vi "KGN Get Pump Massflow.vi"(7 "scaling":dbl=1000000.0, 8 "Fehler (Eingang, kein Fehler)":errorcluster, 9 "Info Cluster":T2, 10 "VISA-Referenz (Eingang)":refnum<visa-resource-name>, 11 "device (Eingang)":u32) -> (0 "Fehler (Ausgang)":errorcluster, 1 "Info Cluster out":T2, 2 "VISA-Referenz (Ausgang)":refnum<visa-resource-name>, 3 "dup device (Ausgang)":u32, 4 "Pump MassFlow-Cluster":T1(array[cluster]), 6 "Kommandos gesendet":string)   [LabVIEW 2020, in "Linearisierung v2.lvlib" / "Gasteiler.lvlib" / "HovaCAL_Interface.lvlib" / "KGN.lvlib" / "KGN GUI Get.lvlib"]
uses:
  KGN GUI Get.lvlib
  Controls/Info Cluster.ctl
  get/get.lvlib
  Controls/Controls.lvlib
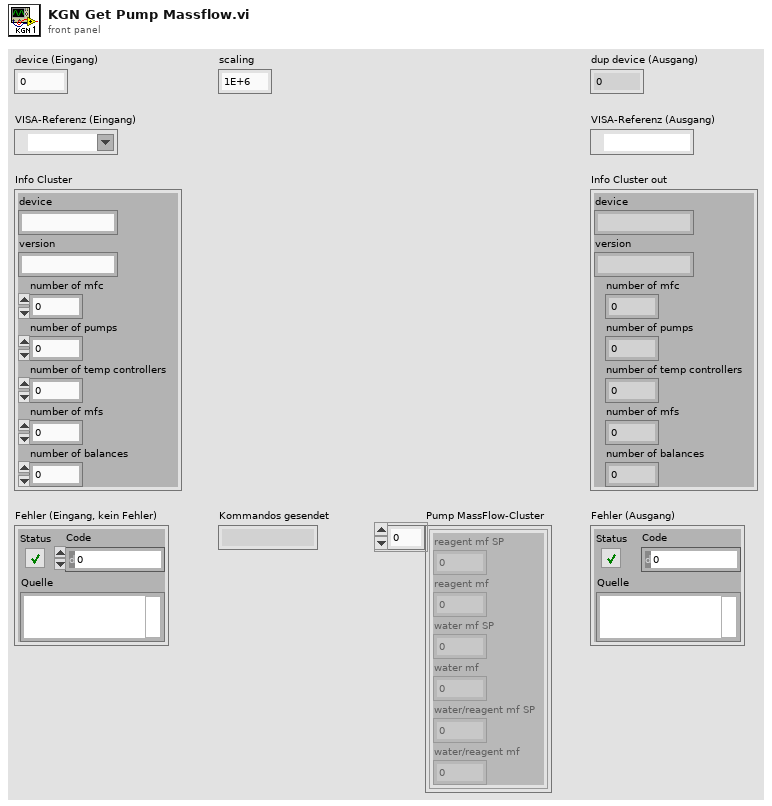
[diagram p1: front panel]
types:
  T1 = cluster{"reagent mf SP":dbl, "reagent mf":dbl, "water mf SP":dbl, "water mf":dbl, "water/reagent mf SP":dbl, "water/reagent mf":dbl}[]
  T2 = typedef "Linearisierung v2.lvlib/Gasteiler.lvlib/HovaCAL_Interface.lvlib/Controls.lvlib/Info Cluster.ctl" = cluster{"device":string, "version":string, "number of mfc":i32, "number of pumps":i32, "number of temp controllers":i32, "number of mfs":i32, "number of balances":i32}
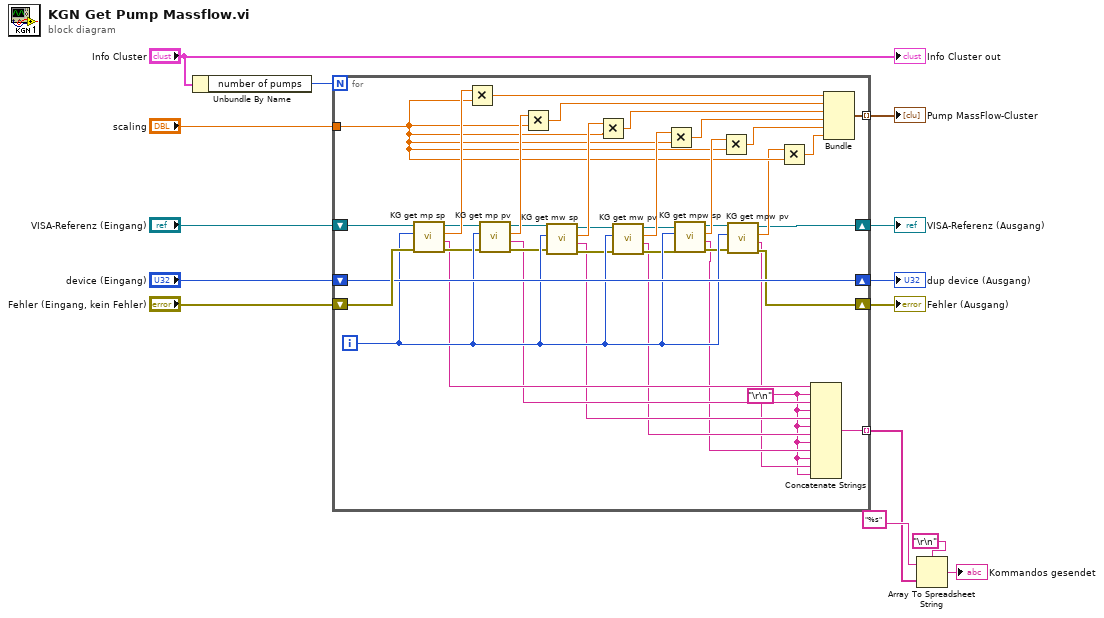
[diagram p0: block diagram]
diagram:
  n1 = Unbundle By Name("Info Cluster") -> ("number of pumps"=w8:i32)
  n2 = for {
    N: w8 -> [_]
    tunnel: [w51] -> w10 mode=indexing
    shift-right: [w50] -> w12
    shift-left: "device (Eingang)" -> [w50]
    shift-right: [w49] -> w11
    shift-left: "Fehler (Eingang, kein Fehler)" -> [w52]
    tunnel: "scaling" -> [w37]
    shift-right: [w33] -> w5
    shift-left: "VISA-Referenz (Eingang)" -> [w34]
    tunnel: [w15] -> w2 mode=indexing
    i -> [w48]
    w16 = "\r\n"
    n3 = call "KG get mp sp.vi"("Fehler (Eingang, kein Fehler)"=w52, "pump"=w48, "VISA-Ressourcenname"=w34) -> ("Fehler (Ausgang)"=w32:errorcluster, "Kommando gesendeet"=w22:string, "Flow"=w47:dbl, "VISA-Ressourcenname (Ausgang)"=w31:refnum<visa-resource-name>)  [unwired: 5 in]
    n4 = Multiply(x=w47, y=w37) -> (x*y=w46:dbl)
    n5 = call "KG get mp pv.vi"("Fehler (Eingang, kein Fehler)"=w32, "pump"=w48, "VISA-Ressourcenname"=w31) -> ("Fehler (Ausgang)"=w29:errorcluster, "Kommando gesendet"=w21:string, "Flow"=w45:dbl, "VISA-Ressourcenname (Ausgang)"=w30:refnum<visa-resource-name>)  [unwired: 5 in]
    n6 = Multiply(x=w45, y=w37) -> (x*y=w44:dbl)
    n7 = call "KG get mw sp.vi"("Fehler (Eingang, kein Fehler)"=w29, "pump"=w48, "VISA-Ressourcenname"=w30) -> ("Fehler (Ausgang)"=w27:errorcluster, "Kommando gesendet"=w20:string, "Flow"=w43:dbl, "VISA-Ressourcenname (Ausgang)"=w28:refnum<visa-resource-name>)  [unwired: 5 in]
    n8 = Multiply(x=w43, y=w37) -> (x*y=w42:dbl)
    n9 = call "KG get mw pv.vi"("Fehler (Eingang, kein Fehler)"=w27, "pump"=w48, "VISA-Ressourcenname"=w28) -> ("Fehler (Ausgang)"=w25:errorcluster, "Kommando gesendet"=w19:string, "Flow"=w41:dbl, "VISA-Ressourcenname (Ausgang)"=w26:refnum<visa-resource-name>)  [unwired: 5 in]
    n10 = Multiply(x=w41, y=w37) -> (x*y=w40:dbl)
    n11 = call "KG get mpw sp.vi"("Fehler (Eingang, kein Fehler)"=w25, "pump"=w48, "VISA-Ressourcenname"=w26) -> ("Fehler (Ausgang)"=w23:errorcluster, "Kommando gesendet"=w18:string, "Flow"=w39:dbl, "VISA-Ressourcenname (Ausgang)"=w24:refnum<visa-resource-name>)  [unwired: 5 in]
    n12 = Multiply(x=w39, y=w37) -> (x*y=w38:dbl)
    n13 = call "KG get mpw pv.vi"("Fehler (Eingang, kein Fehler)"=w23, "pump"=w48, "VISA-Ressourcenname"=w24) -> ("Fehler (Ausgang)"=w49:errorcluster, "Kommando gesendet"=w17:string, "Flow"=w36:dbl, "VISA-Ressourcenname (Ausgang)"=w33:refnum<visa-resource-name>)  [unwired: 5 in]
    n14 = Multiply(x=w36, y=w37) -> (x*y=w35:dbl)
    n15 = Concatenate Strings(w22, w16, w21, w16, w20, w16, w19, w16, w18, w16, w17, w16) -> (w15:string)
    n16 = Bundle(w46, w44, w42, w40, w38, w35) -> (w51:cluster{dbl, dbl, dbl, dbl, dbl, dbl})  [unwired: 1 in]
  }
  "dup device (Ausgang)" <- w12
  "Fehler (Ausgang)" <- w11
  "Pump MassFlow-Cluster" <- w10
  "VISA-Referenz (Ausgang)" <- w5
  n17 = Array To Spreadsheet String(delimiter (Tab)="\r\n", array=w2, 3:"%s" ("Format-String")) -> (spreadsheet string=→"Kommandos gesendet":string)
  "Info Cluster out" <- "Info Cluster"
